vi "Add Vec3d.vi"(8 "error in (no error)":errorcluster, 10 "Vec3d Class in":refnum<class "Vec3d Class.lvclass">, 11 "Vec3d Class in":refnum<class "Vec3d Class.lvclass">) -> (0 "error out":errorcluster, 3 "Vec3d Class out":refnum<class "Vec3d Class.lvclass">)   [LabVIEW 2011, in "Vec3d Class.lvclass"]
uses:
  Vec3d Class.lvclass
  Vec3d Class.lvclass/Vec3d Class.ctl
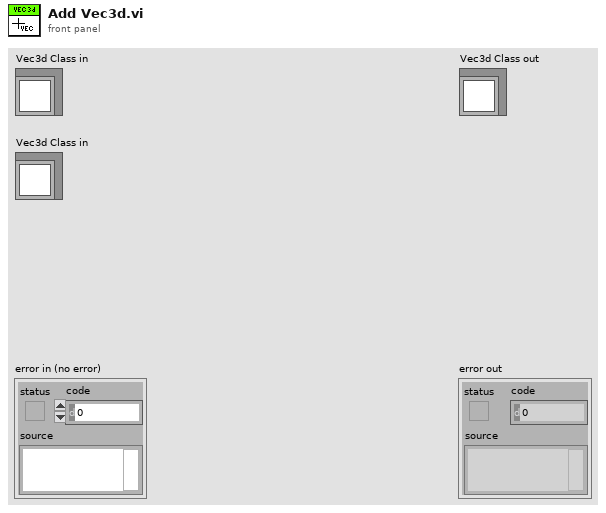
[diagram p1: front panel]
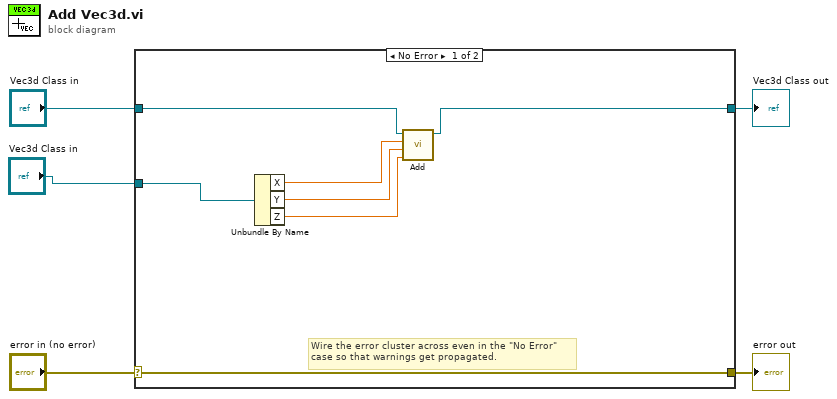
[diagram p0: block diagram]
diagram:
  n1 = case shown="No Error" "error in (no error)" {
    selector: "error in (no error)" -> [w12 w14]
    tunnel: [w12 w14] -> w4
    tunnel: [w10 w13] -> w2
    tunnel: "Vec3d Class in" -> [w11 w13]
    tunnel: "Vec3d Class in" -> [w9 _]
    frame No Error {
      # "Wire the error cluster across even in the \"No Error\"\ncase so that warnings get propagated."
      n2 = Unbundle By Name(w9) -> ("X"=w8:dbl, "Y"=w7:dbl, "Z"=w6:dbl)
      n3 = call-dynamic "Add.vi"("Z"=w6, "Y"=w7, "X"=w8, "Vec3d Class in"=w11) -> ("Vec3d Class out"=w10:refnum<class "Vec3d Class.lvclass">)  [unwired: 7 in]
    }
    frame Error {
    }
  }
  "error out" <- w4
  "Vec3d Class out" <- w2
